vi "Actor Core.vi"(8 "error in":errorcluster, 11 "ServiceManager in":refnum<class "ServiceManager.lvclass">) -> (0 "error out":errorcluster, 3 "Actor out":refnum<class "Actor.lvclass">)   [LabVIEW 2020, in "ServiceManager.lvlib" / "ServiceManager.lvclass"]
doc: "(<B>Filename</B>: Actor Framework.lvlib:Actor.lvclass:Actor Core.vi)\n\nReceives messages to the actor, reacts to them, and initiates any error handling that may shut the actor down.\n\nDescendant classes may override this VI to append parallel tasks for the actor to complete while it handles messages. Overrides use the Call Parent Class Method node."
uses:
  ServiceManager.lvclass
  C:/Program Files (x86)/National Instruments/LabVIEW 2020/vi.lib/ActorFramework/Actor/Actor.lvclass
  <vilib>/ActorFramework/Actor/Actor.lvclass
  ServiceManager.lvclass/ServiceManager.ctl
  Nested/ServiceManager-DebugView/ServiceManager-DebugView/ServiceManager-DebugView.lvclass
  Nested/ServiceManager-Comms/ServiceManager-Comms.lvclass
  C:/Users/taylo/Projects/g-go-service-fwrk/scratchpad/ServiceManagerBeta/ServiceManager/ServiceManager.lvclass
  C:/Users/taylo/Projects/g-go-service-fwrk/scratchpad/ServiceManagerBeta/ServiceManager/Message Handling/Message Handling.lvclass
  C:/Users/taylo/Projects/g-go-service-fwrk/scratchpad/ServiceManagerBeta/ServiceManager/Nested/ServiceManager-DebugView/ServiceManager-DebugView/ServiceManager-DebugView.lvclass
  C:/Users/taylo/Projects/g-go-service-fwrk/scratchpad/ServiceManagerBeta/ServiceManager/Nested/ServiceManager-Comms/ServiceManager-Comms.lvclass
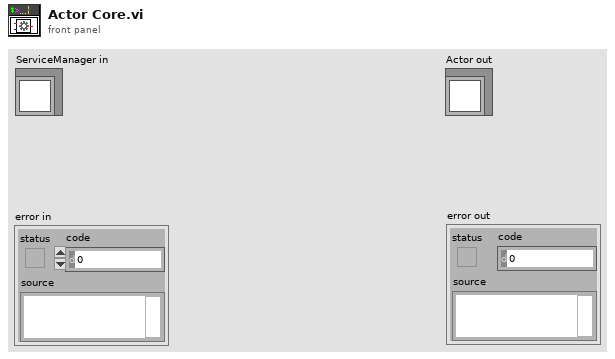
[diagram p1: front panel]
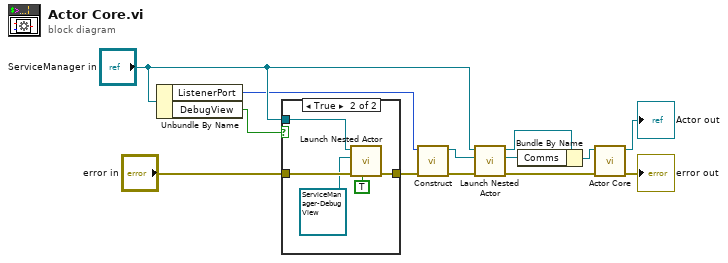
[diagram p0: block diagram]
diagram:
  n1 = Unbundle By Name("ServiceManager in") -> ("ListenerPort"=w2:u16, "DebugView"=w6:bool)
  n2 = case shown="True" w6 {
    tunnel: "ServiceManager in" -> [_ w19]
    tunnel: "error in" -> [w14 w18]
    tunnel: [w14 w16] -> w5
    frame False {
    }
    frame True {
      n3 = call <vilib>:"Launch Nested Actor.vi"("Open Actor Core front panel? (F)"=TRUE, "error in (no error)"=w18, "Nested Actor"=refnum<class "ServiceManager-DebugView.lvclass"> refnum ("ServiceManager.lvlib:ServiceManager-DebugView.lvclass"), "Caller Actor in"=w19) -> ("error out"=w16:errorcluster)  [unwired: 5 in, 2 out]
    }
  }
  n4 = call "Construct.vi"("error in (no error)"=w5, "ListenerPort"=w2) -> ("error out"=w4:errorcluster, "ServiceManager-Comms out"=w1:refnum<class "ServiceManager-Comms.lvclass">)  [unwired: 8 in]
  n5 = call <vilib>:"Launch Nested Actor.vi"("error in (no error)"=w4, "Nested Actor"=w1, "Caller Actor in"="ServiceManager in") -> ("error out"=w11:errorcluster, "Nested Actor's Enqueuer"=w8:refnum<class "Message Enqueuer.lvclass">, "Caller Actor out"=w9:refnum<class "ServiceManager.lvclass">)  [unwired: 6 in]
  n6 = Bundle By Name(cluster=w9, "Comms"=w8) -> (w10:refnum<class "ServiceManager.lvclass">)
  n7 = call-parent "Actor Core.vi"("error in"=w11, "Actor in"=w10) -> ("error out"=→"error out":errorcluster, "Actor out"=→"Actor out":refnum<class "Actor.lvclass">)  [unwired: 8 in]
